vi "ep_Zoom Configuration.vi"(7 "block size":i32, 8 "error in (no error)":errorcluster, 9 "demodulation settings":cluster{"enable? (F)":bool, "algorithm":T4}, 10 "fs":dbl, 11 "spectra settings":T3={"number of lines"=12501, "% overlap"=0.0, "maximum frequency [Hz]"=250.0}) -> (0 "error out":errorcluster, 1 "highpass IIR Filter":T1, 2 "Hilbert FIR filter":cluster{"coefficients":dbl[], "delay":i32}, 3 "zoom FFT settings":T2 {"FFT settings"."window" items=["Rectangle"=0, "Hanning"=1, "Hamming"=2, "Blackman-Harris"=3, "Exact Blackman"=4, "Blackman"=5, "Flat Top"=6, "4 Term B-Harris "=7, "7 Term B-Harris"=8, "Low Sidelobe"=9, "Blackman Nuttall"=11, "Triangle"=30, "Bartlett-Hanning"=31, "Bohman"=32, "Parzen"=33, "Welch"=34, "Kaiser"=60, "Dolph-Chebyshev"=61, "Gaussian"=62]})   [LabVIEW 2014, in "NI_EP_Motor Monitoring.lvlib"]
uses:
  <vilib>/addons/Electrical Power/Motor Monitoring/NI_EP_Motor Monitoring.lvlib
  <vilib>/addons/Electrical Power/Motor Monitoring/subVIs/ep_Demodulation Algorithm.ctl
  <vilib>/addons/Electrical Power/Motor Monitoring/subVIs/ep_Spectra Settings.ctl
  <vilib>/addons/Electrical Power/Motor Monitoring/subVIs/ep_Zoom FFT Settings.ctl
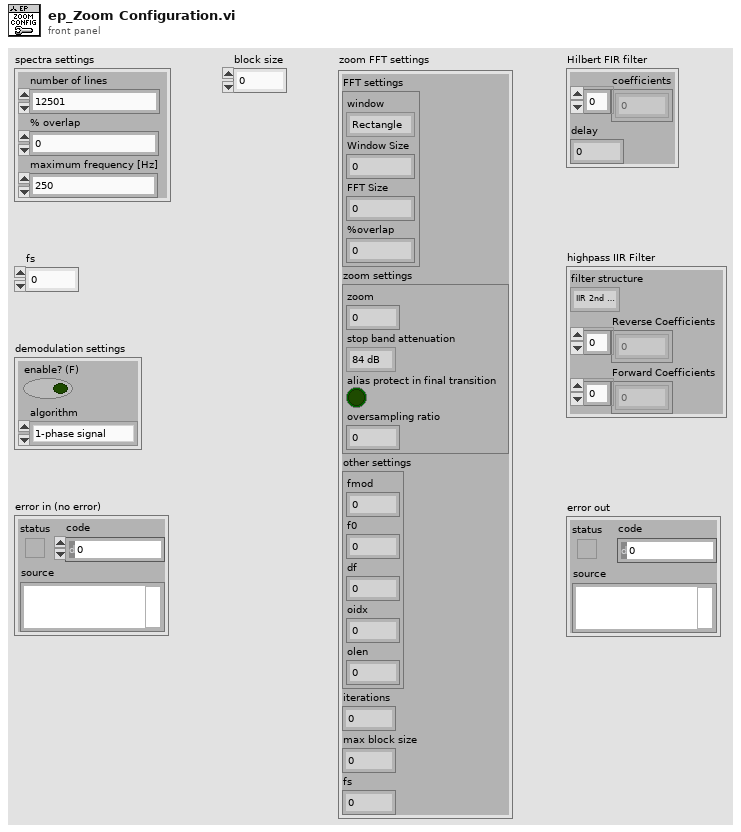
[diagram p1: front panel]
types:
  T1 = cluster{"filter structure":enum32{"IIR 2nd Order", "IIR 4th Order"}, "Reverse Coefficients":dbl[], "Forward Coefficients":dbl[]}
  T2 = typedef "NI_EP_Motor Monitoring.lvlib/ep_Zoom FFT Settings.ctl" = cluster{"FFT settings":cluster{"window":u16, "Window Size":i32, "FFT Size":i32, "%overlap":dbl}, "zoom settings":cluster{"zoom":i32, "stop band attenuation":enum16{"84 dB", "96 dB", "120 dB"}, "alias protect in final transition":bool, "oversampling ratio":dbl}, "other settings":cluster{"fmod":dbl, "f0":dbl, "df":dbl, "oidx":i32, "olen":i32}, "iterations":i32, "max block size":i32, "fs":dbl}
  T3 = typedef "NI_EP_Motor Monitoring.lvlib/ep_Spectra Settings.ctl" = cluster{"number of lines":i32, "% overlap":dbl, "maximum frequency [Hz]":dbl}
  T4 = typedef "NI_EP_Motor Monitoring.lvlib/ep_Demodulation Algorithm.ctl" = enum16{"1-phase signal", "3-phase signals"}
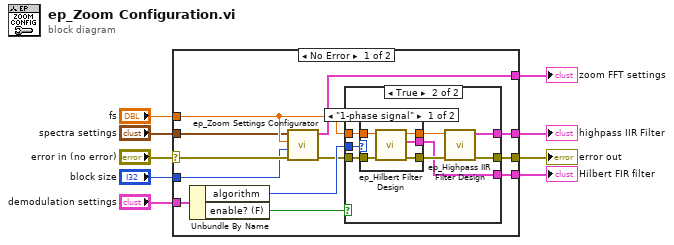
[diagram p0: block diagram]
diagram:
  n1 = case shown="No Error" "error in (no error)" {
    selector: "error in (no error)" -> [w18 w38]
    tunnel: "demodulation settings" -> [w21 _]
    tunnel: "fs" -> [w17 _]
    tunnel: "block size" -> [w16 _]
    tunnel: "spectra settings" -> [w15 _]
    tunnel: [w14 w38] -> w3
    tunnel: [w12 _] -> w4
    tunnel: [w11 _] -> w2
    tunnel: [w10 _] -> w1
    frame No Error {
      n2 = Unbundle By Name(w21) -> ("algorithm"=w20:T4, "enable? (F)"=w19:bool)
      n3 = call <vilib>:"ep_Zoom Settings Configurator.vi"("error in (no error)"=w18, "block size"=w16, "fs"=w17, "spectra settings"=w15) -> ("error out"=w13:errorcluster, "zoom FFT settings"=w12:T2)  [unwired: 6 in]
      n4 = case shown="True" w19 {
        tunnel: w13 -> [w22 w30]
        tunnel: [w22 w25] -> w14
        tunnel: w17 -> [_ w29]
        tunnel: w20 -> [_ w28]
        tunnel: [_ w24] -> w11
        tunnel: [_ w23] -> w10
        frame False {
        }
        frame True {
          n5 = case shown="\"1-phase signal\"" w28 {
            tunnel: w30 -> [w35 w37]
            tunnel: [w34 w37] -> w26
            tunnel: w29 -> [w33 w36]
            tunnel: [w32 w36] -> w27
            tunnel: [w31 _] -> w23
            frame "1-phase signal" {
              n6 = call <vilib>:"ep_Hilbert Filter Design.vi"("error in (no error)"=w35, "fs"=w33) -> ("error out"=w34:errorcluster, "Hilbert FIR filter"=w31:cluster{"h":dbl[], "delay":i32}, "dup fs"=w32:dbl)  [unwired: 7 in]
            }
            frame "3-phase signals", Default {
            }
          }
          n7 = call <vilib>:"ep_Highpass IIR Filter Design.vi"("error in (no error)"=w26, "fs"=w27) -> ("error out"=w25:errorcluster, "highpass IIR Filter"=w24:T1)  [unwired: 8 in]
        }
      }
    }
    frame Error {
    }
  }
  "error out" <- w3
  "zoom FFT settings" <- w4
  "highpass IIR Filter" <- w2
  "Hilbert FIR filter" <- w1
